vi "ProgressPopupWithStatus_Show.vi"(7 "Deployment Notifiers":T1, 8 "error in":errorcluster, 9 "Title":string, 10 "Message":string) -> (0 "error out":errorcluster)   [LabVIEW 2014, in "hse-ui.lvlib"]
doc: "Shows a modal window with an animated progress bar, indicating that some (background) process is running.\n\nThe <b>Title</b> of the window and the <b>Message</b> being displayed can be specified.\n\n\n\n____\nHAMPEL SOFTWARE ENGINEERING v0.7.0 (2018-07-16 18:12)"
uses:
  hse-ui.lvlib
  ProgressPopupWithStatus_Notifiers.ctl
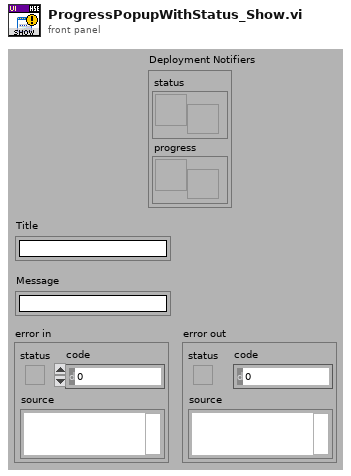
[diagram p1: front panel]
types:
  T1 = typedef "hse-ui.lvlib/ProgressPopupWithStatus_Notifiers.ctl" = cluster{"status":refnum<notifier>, "progress":refnum<notifier>}
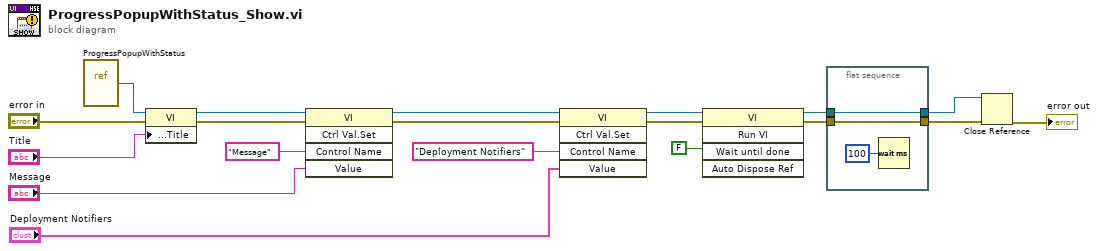
[diagram p0: block diagram]
diagram:
  n1 = vi-ref "ProgressPopupWithStatus.vi"() -> (w8:refnum<vi>)
  n2 = property class="VI"(reference=w8, error in="error in", "Front Panel.Title"="Title") -> (reference out=w15:refnum<vi>, error out=w16:errorcluster)
  n3 = invoke class="VI" method="Ctrl Val.Set"(reference=w15, error in=w16, "Control Name"="Message", "Value"="Message") -> (reference out=w4:refnum<vi>, error out=w3:errorcluster)  [unwired: 1 in, 3 out]
  n4 = invoke class="VI" method="Ctrl Val.Set"(reference=w4, error in=w3, "Control Name"="Deployment Notifiers", "Value"="Deployment Notifiers") -> (reference out=w2:refnum<vi>, error out=w1:errorcluster)  [unwired: 1 in, 3 out]
  n5 = invoke class="VI" method="Run VI"(reference=w2, error in=w1, "Wait until done"=FALSE ("Wait Until Done")) -> (reference out=w12:refnum<vi>, error out=w10:errorcluster)  [unwired: 2 in, 3 out]
  n6 = flat-sequence {
    tunnel: [w22] -> w11
    tunnel: w12 -> [w22]
    tunnel: [w21] -> w9
    tunnel: w10 -> [w21]
    frame #0 {
      n7 = Wait (ms)(milliseconds to wait=u32 100) -> ()  [unwired: 1 out]
    }
  }
  n8 = Close Reference(reference=w11, error in (no error)=w9) -> (error out=→"error out":errorcluster)
